vi "Blink Ready to Drive Indicator.vi"(7 "timeout":i32=1000, 8 "error in":errorcluster, 10 "Dashboard Control in":T1={"Tractive System"=TRUE, "RTD"=TRUE, "AMS error"=TRUE, "IMD error"=TRUE, "Low Voltage"=0.0, "High Voltage"=0.0} {"High Voltage" scale=0.0..10.0; "Low Voltage" scale=0.0..10.0}, 11 "CAN Session In":T2) -> (0 "error out":errorcluster, 2 "Dashboard Control out":T1={"Tractive System"=TRUE, "RTD"=TRUE, "AMS error"=TRUE, "IMD error"=TRUE, "Low Voltage"=0.0, "High Voltage"=0.0} {"High Voltage" scale=0.0..10.0; "Low Voltage" scale=0.0..10.0}, 3 "CAN Session Out":T2)   [LabVIEW 2016]
uses:
  Dashboard Control.ctl
  Program Files (x86)/National Instruments/LabVIEW 2016/examples/robotics/EPOS2 CANOpen Driver/Low Level VIs/Typedefs/CAN Refnum.ctl
  Program Files (x86)/National Instruments/LabVIEW 2016/examples/robotics/EPOS2 CANOpen Driver/Low Level VIs/Typedefs/CAN Session Pointer.ctl
  Program Files (x86)/National Instruments/LabVIEW 2016/examples/robotics/EPOS2 CANOpen Driver/Low Level VIs/Typedefs/CAN Communication References.ctl
  Program Files (x86)/National Instruments/LabVIEW 2016/examples/robotics/EPOS2 CANOpen Driver/Low Level VIs/Typedefs/kill process notifier array.ctl
  Program Files (x86)/National Instruments/LabVIEW 2016/examples/robotics/EPOS2 CANOpen Driver/Low Level VIs/Typedefs/Write Queue.ctl
  Program Files (x86)/National Instruments/LabVIEW 2016/examples/robotics/EPOS2 CANOpen Driver/Low Level VIs/Typedefs/FPGA CAN Frame Cluster.ctl
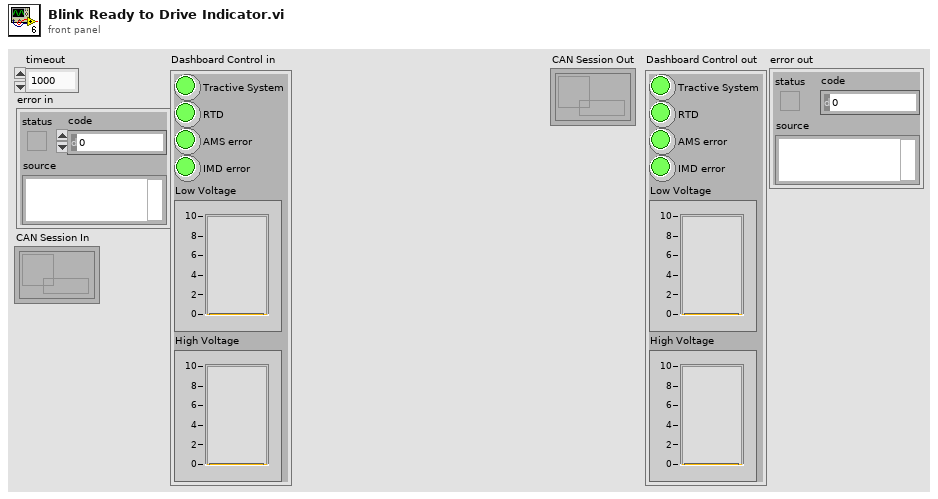
[diagram p1: front panel]
types:
  T1 = typedef "Dashboard Control.ctl" = cluster{"Tractive System":bool, "RTD":bool, "AMS error":bool, "IMD error":bool, "Low Voltage":dbl, "High Voltage":dbl}
  T2 = typedef "CAN Refnum.ctl" = refnum<k1>
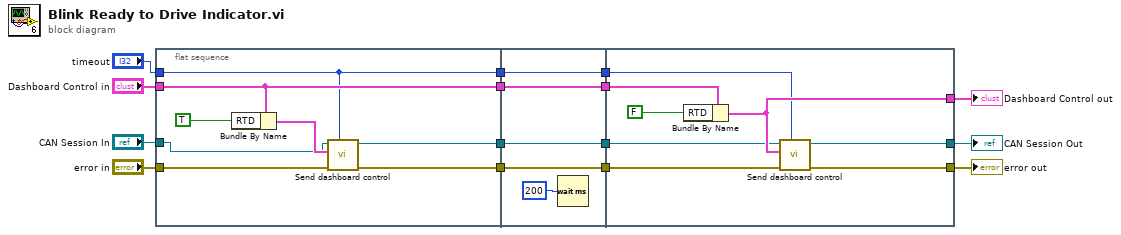
[diagram p0: block diagram]
diagram:
  n1 = flat-sequence {
    tunnel: [w23] -> w14
    tunnel: "Dashboard Control in" -> [w20]
    tunnel: [w20] -> w12
    tunnel: "CAN Session In" -> [w19]
    tunnel: "error in" -> [w18]
    tunnel: [w17] -> w5
    tunnel: [w16] -> w4
    tunnel: "timeout" -> [w16]
    tunnel: [w27] -> w15
    tunnel: w14 -> [w27]
    tunnel: w12 -> [w26]
    tunnel: [w26] -> w11
    tunnel: [w25] -> w6
    tunnel: w5 -> [w25]
    tunnel: w4 -> [w24]
    tunnel: [w24] -> w3
    tunnel: w15 -> [w36]
    tunnel: w11 -> [w35]
    tunnel: [w33] -> w9
    tunnel: [w32] -> w7
    tunnel: w6 -> [w31]
    tunnel: w3 -> [w30]
    tunnel: [w29] -> w2
    frame #0 {
      n2 = Bundle By Name(cluster=w20, "RTD"=TRUE ("Tractive System")) -> (w22:T1)
      n3 = call "Send dashboard control.vi"("timeout"=w16, "error in"=w18, "Dashboard Control"=w22, "CAN Session In"=w19) -> ("error out"=w23:errorcluster, "CAN Session Out"=w17:T2)  [unwired: 6 in]
    }
    frame #1 {
      n4 = Wait (ms)(milliseconds to wait=u32 200) -> ()  [unwired: 1 out]
    }
    frame #2 {
      n5 = Bundle By Name(cluster=w35, "RTD"=FALSE ("Tractive System")) -> (w32:T1)
      n6 = call "Send dashboard control.vi"("timeout"=w30, "error in"=w36, "Dashboard Control"=w32, "CAN Session In"=w31) -> ("error out"=w29:errorcluster, "CAN Session Out"=w33:T2)  [unwired: 6 in]
    }
  }
  "CAN Session Out" <- w9
  "Dashboard Control out" <- w7
  "error out" <- w2
